vi "StateSpaceTester.vi"() -> ()   [LabVIEW 2017]
uses:
  <vilib>/Rock Robotics/WPI/ThirdParty/Phoenix-LabVIEW/Motor Controller/Controls/CTRE_Phoenix_MotorControl_FeedbackDevice.ctl
  <vilib>/Rock Robotics/WPI/ThirdParty/Phoenix-LabVIEW/Motor Controller/Controls/CTRE_Phoenix_MotorControl_LimitSwitchNormal.ctl
  <vilib>/Rock Robotics/WPI/ThirdParty/Phoenix-LabVIEW/Motor Controller/Controls/CTRE_Phoenix_MotorControl_LimitSwitchSource_Local.ctl
  <vilib>/Rock Robotics/WPI/ThirdParty/Phoenix-LabVIEW/Motor Controller/Controls/CTRE_Phoenix_MotorControl_NeutralMode.ctl
  <vilib>/Analysis/Matrix/Datatypes/RealMatrix.ctl
  <vilib>/Rock Robotics/WPI/DriverStation/WPI_DriverStationRobotMode2.ctl
  <vilib>/Rock Robotics/WPI/ThirdParty/Phoenix-LabVIEW/Motor Controller/Controls/CTRE_Phoenix_MotorControl_ControlMode.ctl
  <vilib>/Rock Robotics/WPI/ThirdParty/Phoenix-LabVIEW/Motor Controller/Get/CTRE_Phoenix_MotorController_GetSelectedSensorData.vi
  <vilib>/Analysis/Matrix/NI_Matrix.lvlib
panel:
  in  "Config":T1={"TargetPos"=1.8, "InitalPos"=0.0, "FinalVel"=0.0, "IntitialVel"=0.0, "MaxVel"=2.3, "MaxAccel"=4.0}
  in  "Run again":bool
  in  "Output":dbl(slide)=-2.0 scale=-2.0..2.0
  in  "Manual":bool
  in  "Parameters":T2={"Mass"=12.0, "GearRatio"=24.0, "Radius"=0.025, "Resistance"=0.08, "Ki"=0.0025, "Ke"=0.0045, "Friction"=0.0}
  in  "Reset Sensor":bool
  out "Vel":T3(graph)={0.0, "Real Matrix Element"=0.0005668820410795566, "Real Matrix Element"=0.0}
  out "Pos":T3(graph)={1.799768462219455, "Real Matrix Element"=1.602720144198555, "Real Matrix Element"=1.8}
  in  "GravityCompensator":dbl=1.22 format="%#_13g"
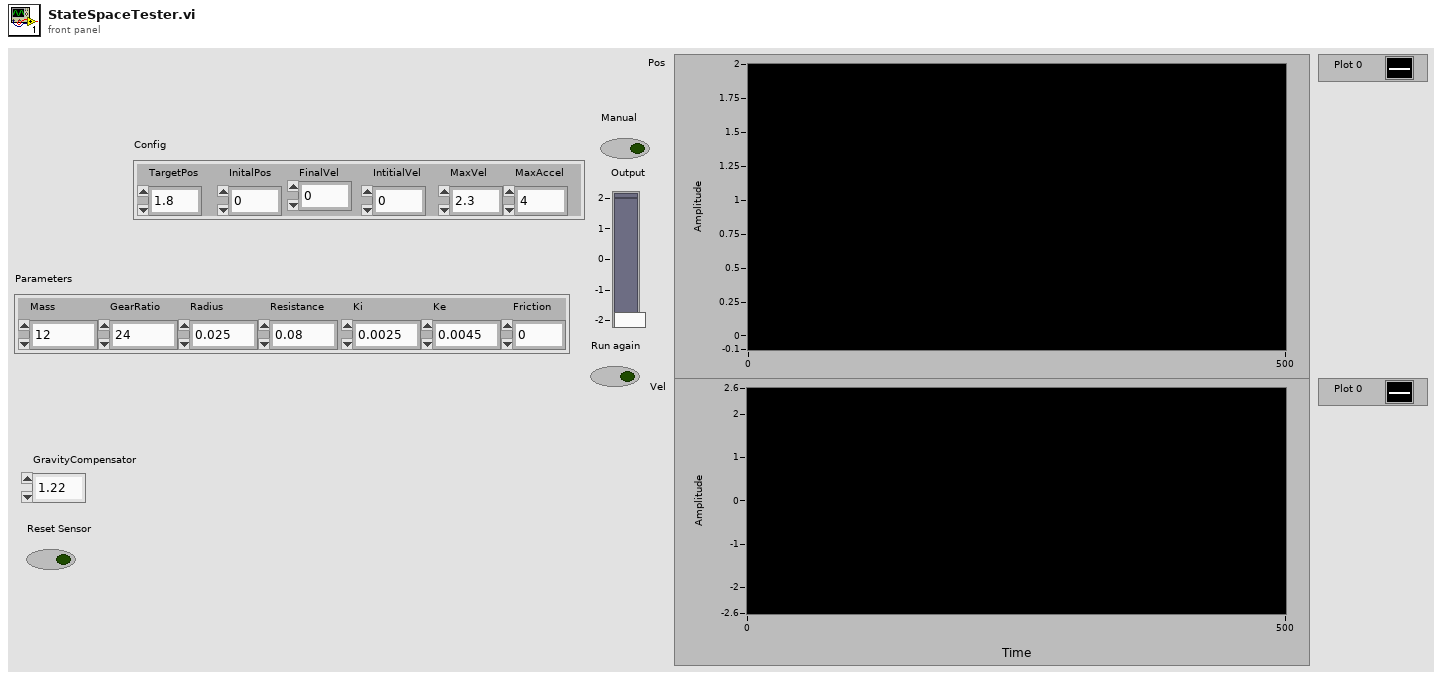
[diagram p1: front panel]
types:
  T1 = cluster{"TargetPos":dbl, "InitalPos":dbl, "FinalVel":dbl, "IntitialVel":dbl, "MaxVel":dbl, "MaxAccel":dbl}
  T2 = cluster{"Mass":dbl, "GearRatio":dbl, "Radius":dbl, "Resistance":dbl, "Ki":dbl, "Ke":dbl, "Friction":dbl}
  T3 = cluster{dbl, "Real Matrix Element":dbl, "Real Matrix Element":dbl}
  T4 = typedef "NI_Matrix.lvlib/RealMatrix.ctl" = dbl[][]
  T5 = typedef "CTRE_Phoenix_MotorControl_NeutralMode.ctl" = enum8{"EEPROMSetting", "Override to Coast", "Override to Brake"}
  T6 = typedef "CTRE_Phoenix_MotorControl_LimitSwitchSource_Local.ctl" = enum16{"Feedback Connector", "Remote Talon SRX", "Remote CANifier", "Deactivated"}
  T7 = typedef "CTRE_Phoenix_MotorControl_LimitSwitchNormal.ctl" = enum16{"Normally Open", "Normally Closed", "Disabled"}
  T8 = typedef "CTRE_Phoenix_MotorControl_FeedbackDevice.ctl" = i8
  T9 = typedef "WPI_MotorControlDeviceRef.ctl" = cluster{"DeviceStatus":errorcluster, "Type":T10, "PWM":cluster{"PWM Channel":T11, "DeadBand":T12}, "CAN":cluster{"Device Number":u8, "SetOutput VI Ref":variant, "GetOutput VI Ref":variant, "Enable VI Ref":variant, "Disable VI Ref":variant, "Data":variant}, "Invert":bool, "DIO PWM":cluster{"PWM \"Enable\" Channel":T11, "DIOChannel":T13, "PWM Rate":dbl}}
  T10 = typedef "WPI_MotorControlType.ctl" = enum16{"PWM", "CAN", "DIO PWM"}
  T11 = typedef "FPGA_DIOPWMChannel.ctl" = enum8{"PWM 0", "PWM 1", "PWM 2", "PWM 3", "PWM 4", "PWM 5", "PWM 6", "PWM 7", "PWM 8", "PWM 9", "PWM MXP 0", "PWM MXP 1", "PWM MXP 2", "PWM MXP 3", "PWM MXP 4", "PWM MXP 5", "PWM MXP 6", "PWM MXP 7", "PWM MXP 8", "PWM MXP 9", "Invalid"}
  T12 = typedef "WPI_PWMDeadband.ctl" = cluster{"Name":string, "maxPositivePwm":i32, "minPositivePwm":i32, "centerPwm":i32, "maxNegativePwm":i32, "minNegativePwm":i32, "angularRange":u16}
  T13 = typedef "FPGA_DIOChannel.ctl" = enum8{"DIO 0", "DIO 1", "DIO 2", "DIO 3", "DIO 4", "DIO 5", "DIO 6", "DIO 7", "DIO 8", "DIO 9", "DIO MXP 0", "DIO MXP 1", "DIO MXP 2", "DIO MXP 3", "DIO MXP 4", "DIO MXP 5", "DIO MXP 6", "DIO MXP 7", "DIO MXP 8", "DIO MXP 9", "DIO MXP 10", "DIO MXP 11", "DIO MXP 12", "DIO MXP 13", "DIO MXP 14", "DIO MXP 15", "SPI Port CS1", "SPI Port CS2", "SPI Port CS3", "SPI Port MISO", "SPI Port MOSI", "Invalid"}
  T14 = typedef "WPI_DriverStationRobotMode2.ctl" = enum16{"Autonomous Disabled", "Autonomous Enabled", "Teleop Disabled", "Teleop Enabled", "Disconnected", "Finish", "Test Disabled", "Test Enabled", "Emergency Stopped"}
  T15 = typedef "CTRE_Phoenix_MotorControl_ControlMode.ctl" = u16
  T16 = cluster{"Gains":cluster{"A":T4, "B":T4, "C":T4, "D":T4, "Q":T4, "R":T4, "K":T4, "Kff":T4, "L":T4}, "X":T4}
  T17 = cluster{"A":T4, "B":T4, "C":T4, "D":T4, "Q":T4, "R":T4, "K":T4, "Kff":T4, "L":T4}
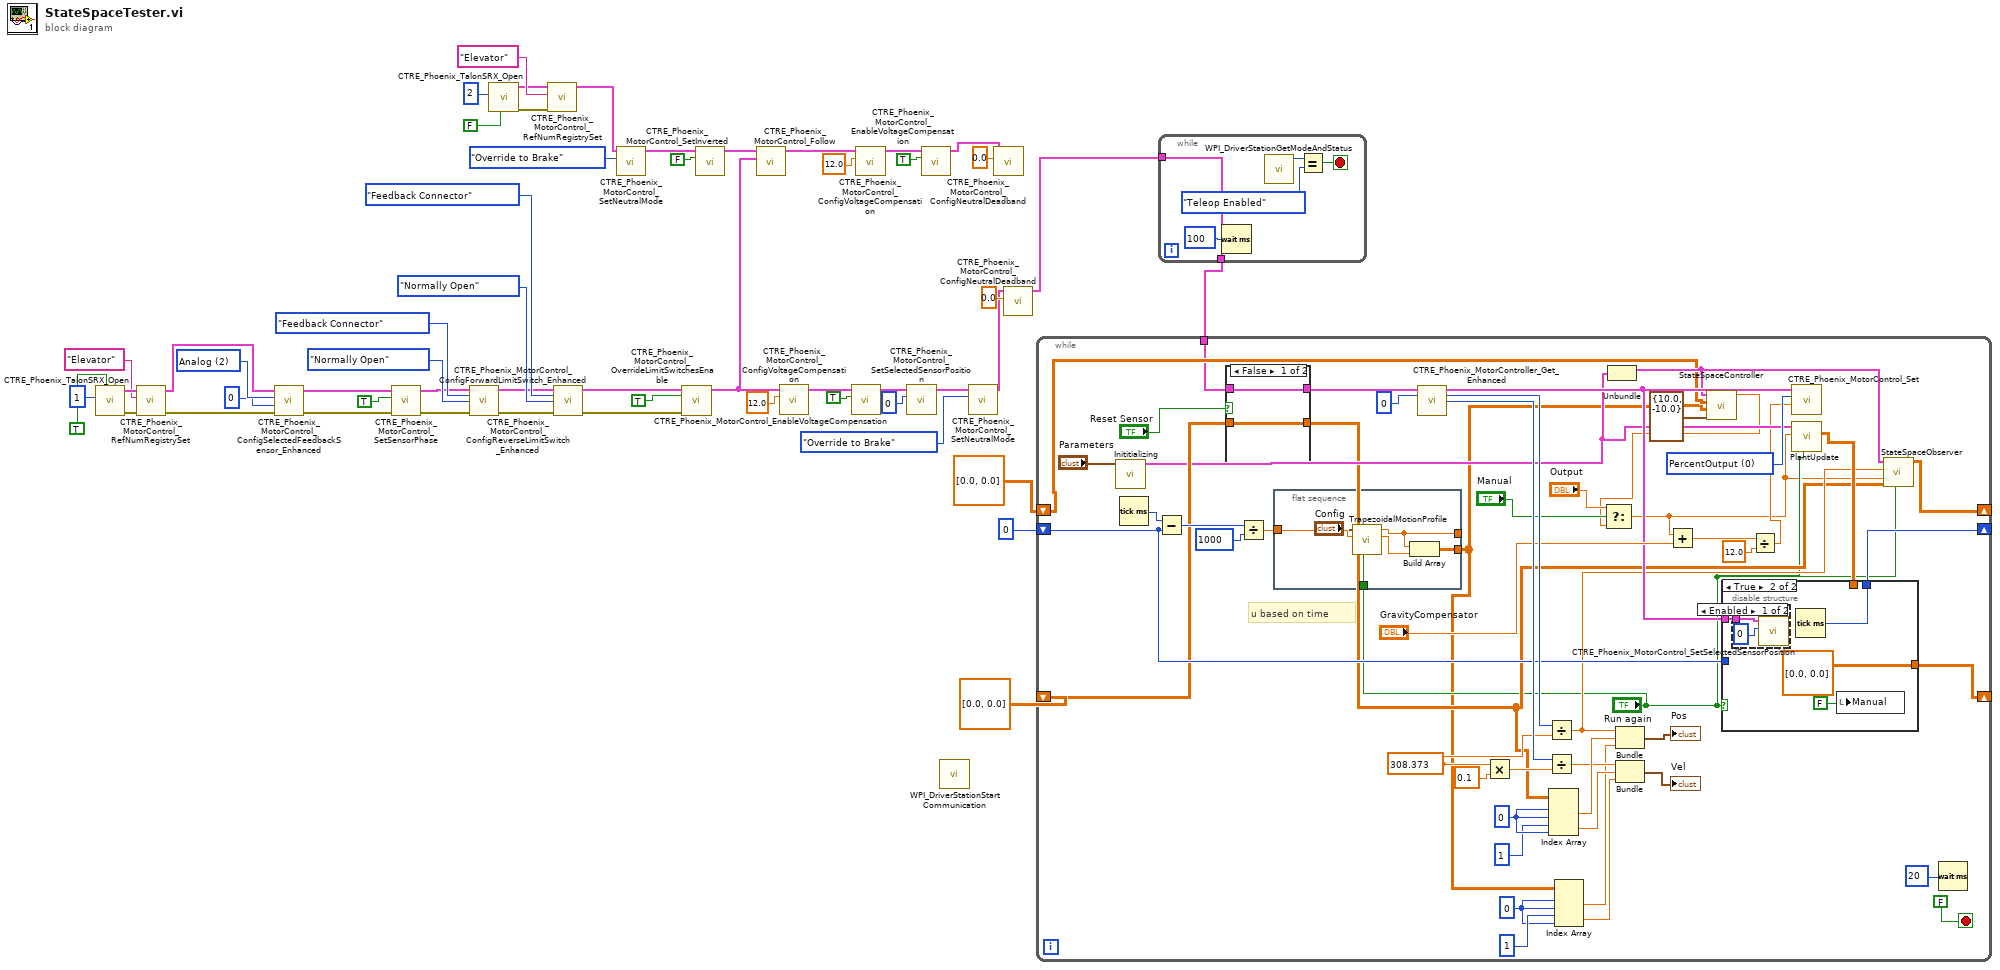
[diagram p0: block diagram]
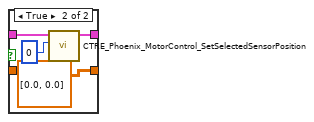
[diagram p4: hidden frame]
diagram:
  w49 = T8 2 items=["None"=-1, "QuadEncoder"=0, "Analog"=2, "Tachometer"=4, "Pulse Width Encoded Position"=8, "Sensor Sum (S0 + S1)"=9, "Sensor Difference (D0 - D1)"=10, "Remote Source 0"=11, "Remote Source 1"=12, "Software Emulated"=15] ("Feedback Device")
  n1 = call <vilib>:"CTRE_Phoenix_TalonSRX_Open.vi"("Invert"=TRUE, "Device Number"=u8 1) -> ("error out"=w53:errorcluster, "CAN Talon SRX Ref"=w54:T9)  [unwired: 8 in]
  n2 = call <vilib>:"CTRE_Phoenix_MotorControl_RefNumRegistrySet.vi"("error in (no error)"=w53, "refnum name"="Elevator", "PhoenixMotorControlDevRef"=w54) -> ("error out"=w50:errorcluster, "PhoenixMotorControlDevRef"=w32:T9)  [unwired: 7 in]
  n3 = call <vilib>:"CTRE_Phoenix_MotorControl_ConfigSelectedFeedbackSensor_Enhanced.vi"("error in (no error)"=w50, "pidLoopIdx"=0, "Feedback Device"=w49, "PhoenixMotorControlDevRef"=w32) -> ("error out"=w29:errorcluster, "PhoenixMotorControlDevRef"=w31:T9)  [unwired: 6 in]
  n4 = call <vilib>:"CTRE_Phoenix_MotorControl_SetSensorPhase.vi"("error in (no error)"=w29, "PhaseSensor"=TRUE, "PhoenixMotorControlDevRef"=w31) -> ("error out"=w28:errorcluster, "PhoenixMotorControlDevRef"=w30:T9)  [unwired: 7 in]
  n5 = call <vilib>:"CTRE_Phoenix_MotorControl_ConfigReverseLimitSwitch_Enhanced.vi"("PhoenixMotorControlDevRef"=w30, "Limit Switch Source"=CTRE_Phoenix_MotorControl_LimitSwitchSource_Local."Feedback Connector", "NormallyOpenOrClosed"=CTRE_Phoenix_MotorControl_LimitSwitchNormal."Normally Open", "error in (no error)"=w28) -> ("PhoenixMotorControlDevRef"=w40:T9, "error out"=w39:errorcluster)  [unwired: 10 in]
  n6 = call <vilib>:"CTRE_Phoenix_TalonSRX_Open.vi"("Invert"=FALSE, "Device Number"=u8 2) -> ("error out"=w36:errorcluster, "CAN Talon SRX Ref"=w35:T9)  [unwired: 8 in]
  n7 = call <vilib>:"CTRE_Phoenix_MotorControl_RefNumRegistrySet.vi"("error in (no error)"=w36, "refnum name"="Elevator", "PhoenixMotorControlDevRef"=w35) -> ("PhoenixMotorControlDevRef"=w25:T9)  [unwired: 7 in, 1 out]
  n8 = call <vilib>:"CTRE_Phoenix_MotorControl_ConfigForwardLimitSwitch_Enhanced.vi"("PhoenixMotorControlDevRef"=w40, "Limit Switch Source"=CTRE_Phoenix_MotorControl_LimitSwitchSource_Local."Feedback Connector", "NormallyOpenOrClosed"=CTRE_Phoenix_MotorControl_LimitSwitchNormal."Normally Open", "error in (no error)"=w39) -> ("PhoenixMotorControlDevRef"=w43:T9, "error out"=w42:errorcluster)  [unwired: 10 in]
  n9 = call <vilib>:"CTRE_Phoenix_MotorControl_SetNeutralMode.vi"("Motor Control Neutral Mode"=CTRE_Phoenix_MotorControl_NeutralMode."Override to Brake", "PhoenixMotorControlDevRef"=w25) -> ("PhoenixMotorControlDevRef"=w22:T9)  [unwired: 8 in, 1 out]
  n10 = call <vilib>:"CTRE_Phoenix_MotorControl_OverrideLimitSwitchesEnable.vi"("PhoenixMotorControlDevRef"=w43, "Override Limit Switch Enable?"=TRUE, "error in (no error)"=w42) -> ("PhoenixMotorControlDevRef"=w14:T9)  [unwired: 11 in, 1 out]
  n11 = call <vilib>:"CTRE_Phoenix_MotorControl_SetInverted.vi"("Invert?"=FALSE, "PhoenixMotorControlDevRef"=w22) -> ("PhoenixMotorControlDevRef"=w11:T9)  [unwired: 8 in, 1 out]
  n12 = call <vilib>:"CTRE_Phoenix_MotorControl_Follow.vi"("Master Controller to Follow"=w14, "PhoenixMotorControlDevRef"=w11) -> ("PhoenixMotorControlDevRef"=w21:T9)  [unwired: 8 in, 1 out]
  n13 = call <vilib>:"CTRE_Phoenix_MotorControl_ConfigVoltageCompensation.vi"("Saturation Voltage"=12.0, "PhoenixMotorControlDevRef"=w14) -> ("PhoenixMotorControlDevRef"=w16:T9)  [unwired: 8 in, 1 out]
  n14 = call <vilib>:"CTRE_Phoenix_MotorControl_EnableVoltageCompensation.vi"("Enable Voltage Compensation?"=TRUE, "PhoenixMotorControlDevRef"=w16) -> ("PhoenixMotorControlDevRef"=w12:T9)  [unwired: 8 in, 1 out]
  n15 = call <vilib>:"CTRE_Phoenix_MotorControl_ConfigVoltageCompensation.vi"("Saturation Voltage"=12.0, "PhoenixMotorControlDevRef"=w21) -> ("PhoenixMotorControlDevRef"=w19:T9)  [unwired: 8 in, 1 out]
  n16 = call <vilib>:"CTRE_Phoenix_MotorControl_SetSelectedSensorPosition.vi"("New Sensor Position"=0, "PhoenixMotorControlDevRef"=w12) -> ("PhoenixMotorControlDevRef"=w10:T9)  [unwired: 8 in, 1 out]
  n17 = call <vilib>:"CTRE_Phoenix_MotorControl_EnableVoltageCompensation.vi"("Enable Voltage Compensation?"=TRUE, "PhoenixMotorControlDevRef"=w19) -> ("PhoenixMotorControlDevRef"=w5:T9)  [unwired: 8 in, 1 out]
  n18 = call <vilib>:"WPI_DriverStationStart Communication.vi"() -> ()  [unwired: 12 in]
  n19 = call <vilib>:"CTRE_Phoenix_MotorControl_SetNeutralMode.vi"("Motor Control Neutral Mode"=CTRE_Phoenix_MotorControl_NeutralMode."Override to Brake", "PhoenixMotorControlDevRef"=w10) -> ("PhoenixMotorControlDevRef"=w6:T9)  [unwired: 8 in, 1 out]
  n20 = call <vilib>:"CTRE_Phoenix_MotorControl_ConfigNeutralDeadband.vi"("Percent Deadband"=0.0, "PhoenixMotorControlDevRef"=w5) -> ()  [unwired: 8 in, 2 out]
  n21 = call <vilib>:"CTRE_Phoenix_MotorControl_ConfigNeutralDeadband.vi"("Percent Deadband"=0.0, "PhoenixMotorControlDevRef"=w6) -> ("PhoenixMotorControlDevRef"=w1:T9)  [unwired: 8 in, 1 out]
  n22 = while {
    tunnel: [w58] -> w2
    tunnel: w1 -> [w58]
    stop <- w55 stop-if-true
    n23 = Wait (ms)(milliseconds to wait=u32 100) -> ()  [unwired: 1 out]
    n24 = call <vilib>:"WPI_DriverStationGetModeAndStatus.vi"() -> ("Robot Mode"=w57:T14)  [unwired: 10 in, 1 out]
    n25 = Equal?(x=w57, y=WPI_DriverStationRobotMode2."Teleop Enabled") -> (x = y?=w55:bool)
  }
  n26 = while {
    shift-right: [w82] -> _
    shift-left: T4 [[0.0], [0.0]] ("X (Not visible on real robot)") -> [w78]
    shift-right: [w83] -> _
    shift-left: u32 0 ("millisecond timer value") -> [w80]
    shift-right: [w71] -> _
    shift-left: T4 [[0.0], [0.0]] ("X (Not visible on real robot)") -> [w70]
    tunnel: w2 -> [w69]
    stop <- FALSE stop-if-true
    w63 = 0 ("index (row)")
    w97 = 0 ("index (row)")
    w92 = 308.373
    w108 = T15 0 items=["PercentOutput"=0, "Position"=1, "Velocity"=2, "Current"=3, "Follower"=5, "MotionProfile"=6, "MotionMagic"=7, "MotionMagicArc"=8, "MotionProfileArc"=10, "Disabled"=15] ("Control Mode")
    # "u based on time"
    n27 = call "Inititializing.vi"("Parameters"="Parameters") -> ("Plant"=w75:T16)  [unwired: 10 in]
    n28 = Tick Count (ms)() -> (millisecond timer value=w103:u32)
    n29 = Subtract(x=w103, y=w80) -> (x-y=w102:u32)
    n30 = case shown="False" "Reset Sensor" {
      tunnel: [w119 w123] -> w86
      tunnel: w78 -> [w120 _]
      tunnel: [w120 T4 [[0.0], [0.0]] ("X (Not visible on real robot)")] -> w72
      tunnel: w69 -> [w119 w121]
      frame False {
      }
      frame True {
        n31 = call <vilib>:"CTRE_Phoenix_MotorControl_SetSelectedSensorPosition.vi"("New Sensor Position"=0, "PhoenixMotorControlDevRef"=w121) -> ("PhoenixMotorControlDevRef"=w123:T9)  [unwired: 8 in, 1 out]
      }
    }
    n32 = Divide(x=w102, y=u32 1000) -> (x/y=w100:dbl)
    n33 = flat-sequence {
      tunnel: w100 -> [w130]
      tunnel: [w127] -> _
      tunnel: [w126] -> w62
      tunnel: "Run again" -> [w125]
      frame #0 {
        n34 = call "TrapezoidalMotionProfile.vi"("Initialize"=w125, "Time"=w130, "Config"="Config") -> ("Velocity"=w128:dbl, "Distance"=w127:dbl)  [unwired: 6 in, 1 out]
        n35 = Build Array(w127, w128) -> (w126:T4)
      }
    }
    n36 = call-poly <vilib>:"CTRE_Phoenix_MotorController_Get_Enhanced.vi"("PhoenixMotorControlDevRef"=w86, "pidLoopIdx"=u32 0) -> ("PhoenixMotorControlDevRef"=w79:T9, "Position (Raw Sensor Units)"=w105:i32, "Velocity (Raw Sensor Units per 100 ms)"=w104:i32)  [unwired: 10 in, 1 out]
    n37 = Multiply(x=w92, y=0.1) -> (x*y=w93:dbl)
    n38 = Divide(x=w105, y=w92) -> (x/y=w73:dbl)
    n39 = Divide(x=w104, y=w93) -> (x/y=w94:dbl)
    n40 = Index Array(array=w72, index (row) #1=w97, index (col) #1=w97, index (row) #2=1 ("index (row)"), index (col) #2=w97) -> (element #1=w95:dbl, element #2=w90:dbl)
    n41 = Index Array(array=w62, index (row) #1=w63, index (col) #1=w63, index (row) #2=1 ("index (row)"), index (col) #2=w63) -> (element #1=w60:dbl, element #2=w61:dbl)
    n42 = Unbundle(w75) -> ("Gains"=w74:T17)  [unwired: 1 out]
    n43 = Bundle(w73, "Real Matrix Element"=w95, "Real Matrix Element"=w60) -> (→"Pos":T3)  [unwired: 1 in]
    n44 = Bundle(w94, "Real Matrix Element"=w90, "Real Matrix Element"=w61) -> (→"Vel":T3)  [unwired: 1 in]
    n45 = call "StateSpaceController.vi"("u_Range"=cluster{"u_max":dbl, "u_min":dbl} {"u_max"=10.0, "u_min"=-10.0}, "goal_next"=w62, "x"=w70, "Gains"=w74) -> ("u"=w67:dbl)  [unwired: 7 in]
    n46 = Select(t="Output", s="Manual", f=w67) -> (s? t:f=w65:dbl)
    n47 = Add(x=w65, y="GravityCompensator") -> (x+y=w98:dbl)
    n48 = Divide(x=w98, y=12.0) -> (x/y=w66:dbl)
    n49 = call <vilib>:"CTRE_Phoenix_MotorControl_Set.vi"("Output"=w66, "Control Mode"=w108, "PhoenixMotorControlDevRef"=w79) -> ()  [unwired: 7 in, 2 out]
    n50 = call "PlantUpdate.vi"("Reinitialize"="Run again", "u"=w65, "Plant"=w75) -> ("X (Not visible on real robot)"=w81:T4)  [unwired: 7 in, 1 out]
    n51 = case shown="True" "Run again" {
      tunnel: [w111 w116] -> w83
      tunnel: [w112 T4 [[0.0], [0.0]] ("X (Not visible on real robot)")] -> w82
      tunnel: w81 -> [w112 _]
      tunnel: w80 -> [w111 _]
      tunnel: w79 -> [_ w115]
      frame False {
      }
      frame True {
        n52 = disable-structure shown="Enabled" {
          disable-tunnel: w115 -> [w117 _]
          frame Enabled {
            n53 = call <vilib>:"CTRE_Phoenix_MotorControl_SetSelectedSensorPosition.vi"("New Sensor Position"=0, "PhoenixMotorControlDevRef"=w117) -> ()  [unwired: 8 in, 2 out]
          }
          frame Disabled {
          }
        }
        n54 = Tick Count (ms)() -> (millisecond timer value=w116:u32)
        n55 = local write "Manual"(FALSE ("Manual")) -> ()
      }
    }
    n56 = call "StateSpaceObserver.vi"("Reinitialize"="Run again", "X_hat_Initial"=w72, "u"=w65, "y"=w73, "Gains"=w74) -> ("X_hat"=w71:T4)  [unwired: 6 in]
    n57 = Wait (ms)(milliseconds to wait=u32 20) -> ()  [unwired: 1 out]
  }
